vi "DBC Get Msg Signal Name.vi"(7 "pSignalName":string, 9 "index":i32, 10 "pMsgName":string, 11 "DBCHandle":u64) -> (2 "pMsgName out":string, 3 "function return":i32, 5 "pSignalName out":string)   [LabVIEW 2010, in "dbc_parser.lvlib"]
doc: "int WINAPI DBC_GetMsgSignalName(long long DBCHandle, char* pMsgName, int index, char* pSignalName);"
uses:
  dbc_parser.lvlib
  USB2XXX/trunk/USB2XXX/USB2XXX/vs2019/Release/USB2XXX.dll
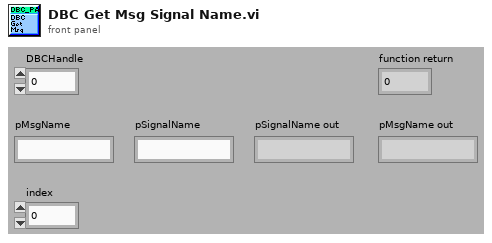
[diagram p1: front panel]
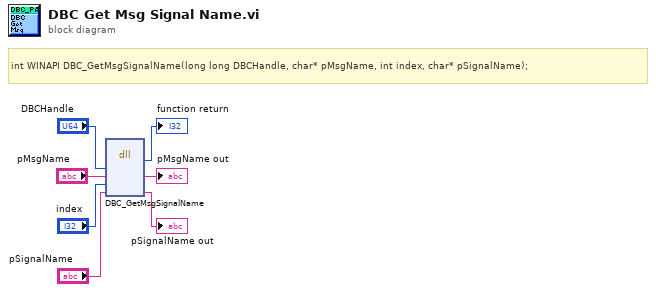
[diagram p0: block diagram]
diagram:
  # "int WINAPI DBC_GetMsgSignalName(long long DBCHandle, char* pMsgName, int index, char* pSignalName);"
  n1 = dll-call lib="E:/Projects/USB2XXX/trunk/USB2XXX/USB2XXX/vs2019/Release/USB2XXX.*" fn="DBC_GetMsgSignalName"("DBCHandle"="DBCHandle", "pMsgName"="pMsgName", "index"="index", "pSignalName"="pSignalName") -> (→"function return":i32, "pMsgName"=→"pMsgName out":string, "pSignalName"=→"pSignalName out":string)  [unwired: 5 in, 2 out]
